vi "Pre Launch Init.vi"(11 "Console Logger in":refnum<class "Console Logger.lvclass">) -> (0 "error out":errorcluster, 3 "Console Logger out":refnum<class "Console Logger.lvclass">)   [LabVIEW 2020, in "Logging.lvlib" / "Console Logger.lvclass"]
doc: "(<B>Filename</B>: Actor Framework.lvlib:Actor.lvclass:Pre Launch Init.vi)\n\nDefines behavior that occurs after the Launch Nested Actor method is invoked but before the actor's Actor Core method begins running.\n\nBy default, this method does nothing. A descendant class may override it to define behavior."
uses:
  Console Logger.lvclass
  Generic Logger/Generic Logger.lvclass
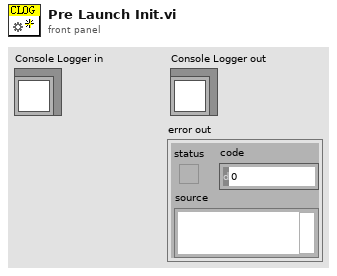
[diagram p1: front panel]
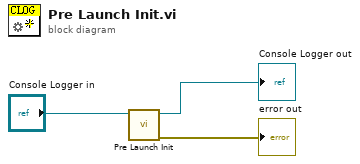
[diagram p0: block diagram]
diagram:
  n1 = call-parent "Pre Launch Init.vi"("Logger in"="Console Logger in") -> ("error out"=→"error out":errorcluster, "Logger out"=→"Console Logger out":refnum<class "Console Logger.lvclass">)  [unwired: 9 in]
